vi "Main.vi"() -> ()   [LabVIEW 2019]
uses:
  Status Image.ctl
  Tile State.ctl
panel:
  out "Opponent's Board":T1[][](array[typedef])
  out "My Board":T1[][](array[typedef])
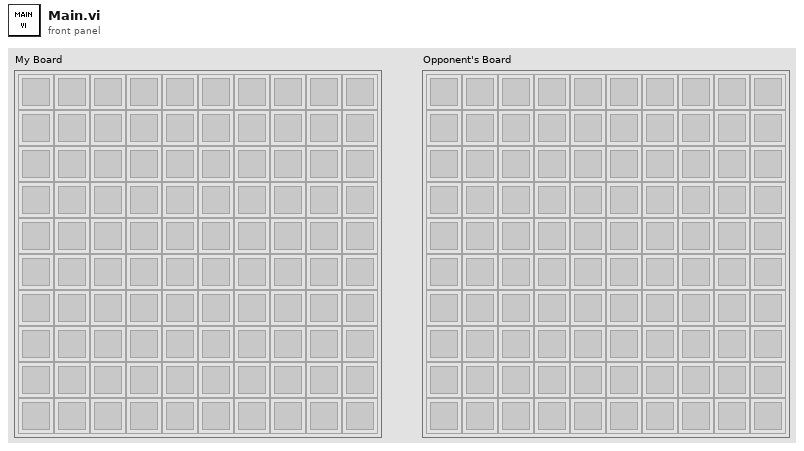
[diagram p1: front panel]
types:
  T1 = typedef "Status Image.ctl" = u16
  T2 = typedef "Tile State.ctl" = enum16{"Unknown", "Empty Water", "My Ship (Hidden)", "My Ship (Hit)", "Opponent's Ship (Revealed)", "Oponnent's Ship (Hit)", "Tentative Location"}
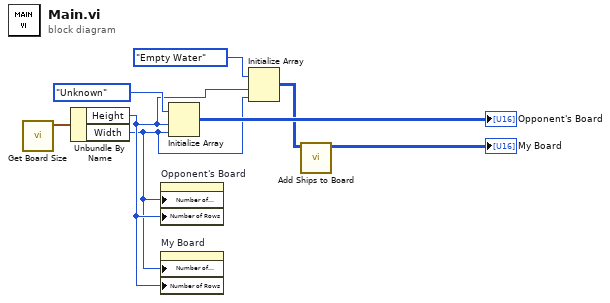
[diagram p0: block diagram]
diagram:
  n1 = call "Get Board Size.vi"() -> ("Board Size"=w8:cluster{"Width":u32, "Height":u32})  [unwired: 11 in]
  n2 = Unbundle By Name(w8) -> ("Height"=w3:u32, "Width"=w2:u32)
  n3 = property on="Opponent's Board" class="Arr (strict)"("Number of Columns"=w2, "Number of Rows"=w3) -> ()  [unwired: 2 in, 2 out]
  n4 = property on="My Board" class="Arr (strict)"("Number of Columns"=w2, "Number of Rows"=w3) -> ()  [unwired: 2 in, 2 out]
  n5 = Initialize Array(Tile_State."Unknown" ("Tile State"), w3, w2) -> (→"Opponent's Board":T2[][])
  n6 = Initialize Array(Tile_State."Empty Water" ("Tile State"), w3, w2) -> (w1:T2[][])
  n7 = call "Add Ships to Board.vi"("Empty Board"=w1) -> ("My Board"=→"My Board":T2[][])  [unwired: 10 in]
